vi "encodeArrayNil.vi"(3 "Boolean Array":bool[](array[boolean])) -> (1 "MessagePack":u8[](array[numeric]) format="%.0x")   [LabVIEW 2015]
uses:
  MsgPackSpeed.lvlib
  encodeBoolean.vi
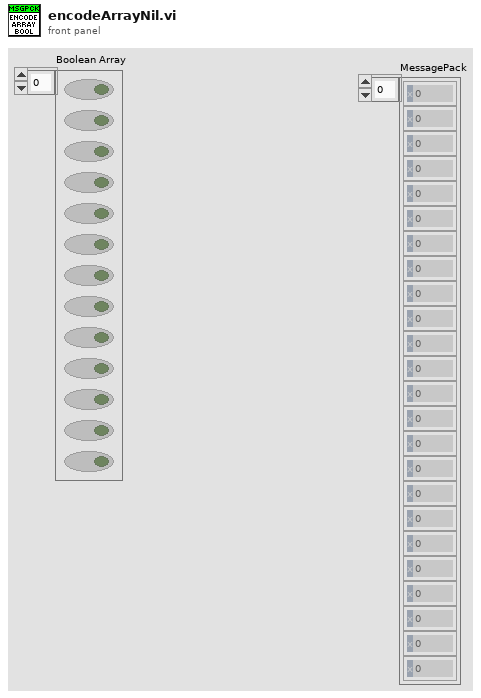
[diagram p1: front panel]
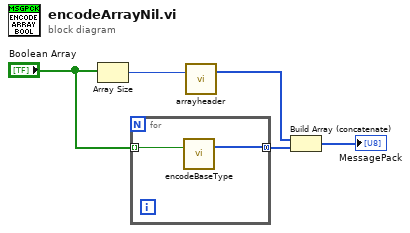
[diagram p0: block diagram]
diagram:
  n1 = Array Size(array="Boolean Array") -> (size(s)=w4:i32)
  n2 = for {
    tunnel: "Boolean Array" -> [w7] mode=indexing
    tunnel: [w6] -> w1 mode=concatenating
    n3 = call-poly "encodeBaseType.vi"("Boolean"=w7) -> ("MessagePack"=w6:u8[])  [unwired: 2 in]
  }
  n4 = call "arrayheader.vi"("Number of Elements"=w4) -> ("header"=w3:u8[])  [unwired: 2 in]
  n5 = Build Array (concatenate)(w3, w1) -> (→"MessagePack":u8[])
